vi "AssertComplex_Image.vi"(8 "error in":errorcluster, 11 "Image Reference In":T1) -> (0 "error out":errorcluster, 3 "Image Reference Out":T1)   [LabVIEW 2020, in "OpenLvVision_OpenCv.lvlib"]
uses:
  OpenLvVision_OpenCv.lvlib
  <vilib>/OpenLvVision/OpenLvVision_Image/Management/TypeDef/OLV ImageType.ctl
  <vilib>/OpenLvVision/OpenLvVision_Image/Management/OLV Management.lvlib
  <vilib>/ErrorRing/Error Ring.xnode
  <vilib>/Utility/error.llb/Error Cluster From Error Code.vi
  <vilib>/OpenLvVision/OpenLvVision_Image/Management/TypeDef/OLV Image.ctl
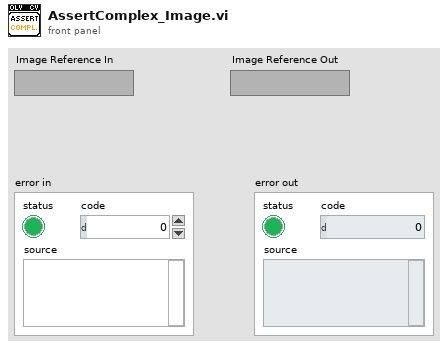
[diagram p1: front panel]
types:
  T1 = typedef "OLV OpenLvVision_Image.lvlib/OLV Management.lvlib/OLV Image.ctl" = refnum<image>
  T2 = typedef "OLV OpenLvVision_Image.lvlib/OLV Management.lvlib/OLV ImageType.ctl" = enum16{"Mono U8", "Mono U16", "Mono I16", "Mono SGL", "Color U32", "Color U64", "Complex CSG"}
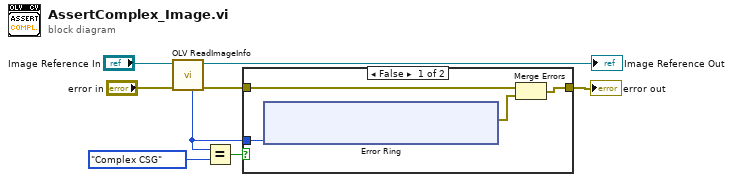
[diagram p0: block diagram]
diagram:
  n1 = call <vilib>:"OLV ReadImageInfo.vi"("error in"="error in", "Image Reference In"="Image Reference In") -> ("error out"=w6:errorcluster, "Image Reference Out"=→"Image Reference Out":T1, "Image Type"=w5:T2)  [unwired: 4 in, 3 out]
  n2 = Equal?(x=w5, y=OLV_ImageType."Complex CSG") -> (x = y?=w7:bool)
  n3 = case shown="False" w7 {
    tunnel: w6 -> [w12 w20]
    tunnel: [w11 w20] -> w3
    tunnel: w5 -> [w9 _]
    frame False {
      n4 = xnode "Error Ring"("parameter 0"=w9) -> ("error out"=w10:errorcluster)
      n5 = Merge Errors(w12, w10) -> (w11:errorcluster)
    }
    frame True {
    }
  }
  "error out" <- w3
